vi "WriteToSensor.vi"(8 "error in (no error)":errorcluster, 11 "SiemensDigitalEnergyMeter in":refnum<class "SiemensDigitalEnergyMeter.lvclass">) -> (0 "error out":errorcluster, 3 "SiemensDigitalEnergyMeter out":refnum<class "SiemensDigitalEnergyMeter.lvclass">)   [LabVIEW 2018, in "SensorPlugins.lvlib" / "SiemensDigitalEnergyMeter.lvclass"]
doc: "This VI sends the provided configuration to the sensor for configuration"
uses:
  SiemensDigitalEnergyMeter.lvclass
  <vilib>/NI/Modbus Library/API/Master/Modbus Master.lvclass
panel:
  out "Test (Did Write to All)":bool
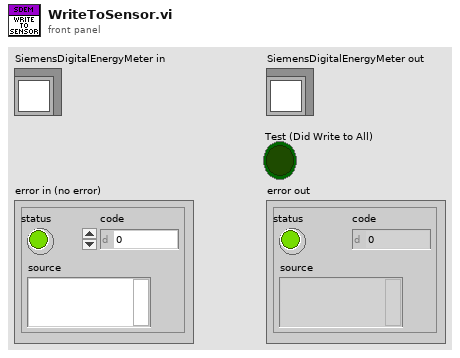
[diagram p1: front panel]
types:
  T1 = typedef "SensorPlugins.lvlib/SiemensDigitalEnergyMeter.lvclass/CommunicationControls.ctl" = refnum<class "Modbus Master.lvclass">[]
  T2 = typedef "SensorPlugins.lvlib/SiemensDigitalEnergyMeter.lvclass/SiemensDigitalEnergyMeterControls.ctl" = cluster{"Measurement(s)":u16[], "Configuration Commands":string, "Use Measurement Commands Text Box?":bool, "Measurement Commands":string, "Connected?":bool, "Serial Number":string, "IP Address":string, "Port (502)":u16, "Unit ID":u8, "Serial Type":enum16{"RTU", "ASCII"}, "Using TCP?":bool, "VISA Resource Name":string}[]
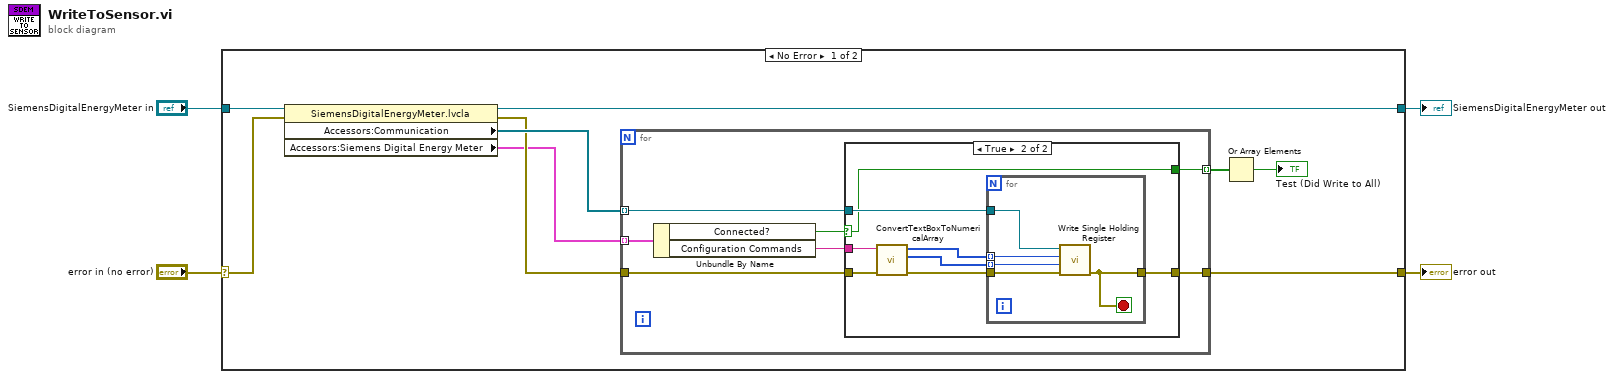
[diagram p0: block diagram]
diagram:
  n1 = case shown="No Error" "error in (no error)" {
    selector: "error in (no error)" -> [w11 w36]
    tunnel: [w8 w36] -> w3
    tunnel: [w12 w35] -> w1
    tunnel: "SiemensDigitalEnergyMeter in" -> [w13 w35]
    frame No Error {
      n2 = property class="SiemensDigitalEnergyMeter.lvcla"(reference=w13, error in=w11) -> (reference out=w12:refnum<class "SiemensDigitalEnergyMeter.lvclass">, error out=w9:errorcluster, "Accessors:Communication"=w10:T1, "Accessors:Siemens Digital Energy Meter"=w7:T2)
      n3 = for {
        tunnel: w10 -> [w20] mode=indexing
        tunnel: w7 -> [w17] mode=indexing
        tunnel: w9 -> [w19]
        tunnel: [w18] -> w8
        tunnel: [w14] -> w6 mode=indexing
        n4 = Unbundle By Name(w17) -> ("Connected?"=w15:bool, "Configuration Commands"=w16:string)
        n5 = case shown="True" w15 {
          selector: w15 -> [_ w22]
          tunnel: w20 -> [_ w29]
          tunnel: w19 -> [w21 w28]
          tunnel: [w21 w24] -> w18
          tunnel: w16 -> [_ w23]
          tunnel: [_ w22] -> w14
          frame False {
          }
          frame True {
            n6 = call "ConvertTextBoxToNumericalArray.vi"("Error In"=w28, "Configuration Commands"=w23) -> ("Error Out"=w27:errorcluster, "Register Value"=w26:u16[], "Register"=w25:u16[])  [unwired: 7 in]
            n7 = for {
              tunnel: w26 -> [w32] mode=indexing
              tunnel: w25 -> [w31] mode=indexing
              tunnel: w29 -> [w30]
              tunnel: w27 -> [w33]
              tunnel: [w34] -> w24
              stop <- w34 stop-if-true
              n8 = call-dynamic "Write Single Holding Register.vi"("error in"=w33, "register to write"=w32, "address"=w31, "Modbus master in"=w30) -> ("error out"=w34:errorcluster)  [unwired: 6 in, 1 out]
            }
          }
        }
      }
      n9 = Or Array Elements(Boolean array=w6) -> (logical OR=→"Test (Did Write to All)":bool)
    }
    frame Error {
    }
  }
  "error out" <- w3
  "SiemensDigitalEnergyMeter out" <- w1
